vi "Initialize HW.vi"(8 "error in (no error)":errorcluster, 11 "Simulated Camera in":refnum<class "Simulated Camera.lvclass">) -> (0 "error out":errorcluster, 3 "Simulated Camera out":refnum<class "Simulated Camera.lvclass">)   [LabVIEW 2020, in "Simulated Camera.lvclass"]
uses:
  Simulated Camera.lvclass
  Simulated Camera.lvclass/Simulated Camera.ctl
  Camera.lvclass
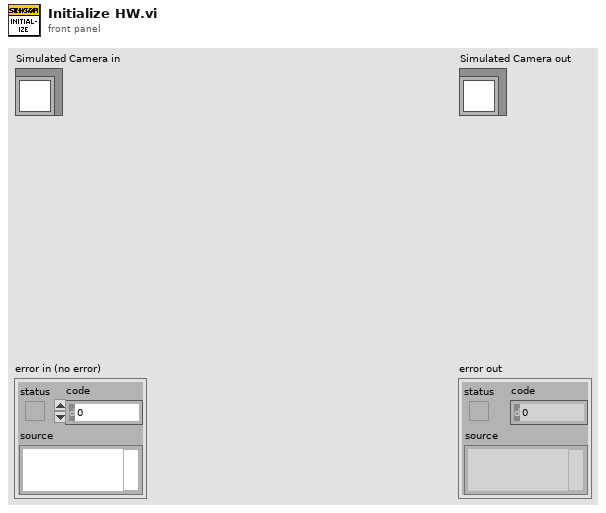
[diagram p1: front panel]
types:
  T1 = enum32{"invalid app kind", "Development System", "Run Time System", "Student Edition", "Embedded LabVIEW", "Evaluation", "Custom"}
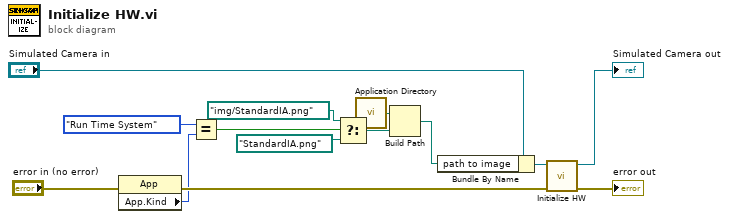
[diagram p0: block diagram]
diagram:
  n1 = property class="App"(error in="error in (no error)") -> (error out=w6:errorcluster, "App.Kind"=w3:T1)  [unwired: 1 in, 1 out]
  n2 = Equal?(x=T1."Run Time System" ("Application:Kind"), y=w3) -> (x = y?=w5:bool)
  n3 = Select(t=path "img/StandardIA.png" ("name or relative path"), s=w5, f=path "StandardIA.png" ("name or relative path")) -> (s? t:f=w2:path)
  n4 = call <vilib>:"Application Directory.vi"() -> ("Application Directory"=w10:path)
  n5 = Build Path(base path=w10, name or relative path=w2) -> (appended path=w1:path)
  n6 = Bundle By Name(cluster="Simulated Camera in", "path to image"=w1) -> (w11:refnum<class "Simulated Camera.lvclass">)
  n7 = call-parent "Initialize HW.vi"("error in (no error)"=w6, "Camera in"=w11) -> ("error out"=→"error out":errorcluster, "Camera out"=→"Simulated Camera out":refnum<class "Simulated Camera.lvclass">)  [unwired: 8 in]
